vi "Register_ValueCalc.vi"(8 "Index":i32, 9 "ADSxxxx Register Data":T1 {"Base" format="%.0x"; "Item Count" format="%.0x"; "Value" format="%.0x"; "RegMap"."Mask" format="%.0x"; "Default" format="%.0x"; "Register" format="%.0x"}, 11 "Register Controls[]":refnum<vi>[](array[refnum])) -> (2 "Register Value Calculated":u32)   [LabVIEW 2010]
doc: "This VI calculates the register value to write based on the current control values. The VI uses the references to the controls to obtain the current value, and sums the shifted values as appropriate for controls location in the configuration register (provide from register map file).\n\nInputs:\nADSxxxx Register Data - (typdef cluster) contains register information parsed from register map text file\nRegister Controls[] - (control ref array) contains control references to all control with a register cluster control\nIndex - (I32) index to replace # in registers that utilize a common typdef (ie CHxSET)\n\nOutputs:\nRegister Value Calculated - (U32) calculated value of configuration register based on current control settings"
uses:
  Scan RegMap/TYP_ADSxxxx Register.ctl
  Scan RegMap/TYP_RegMap Item.ctl
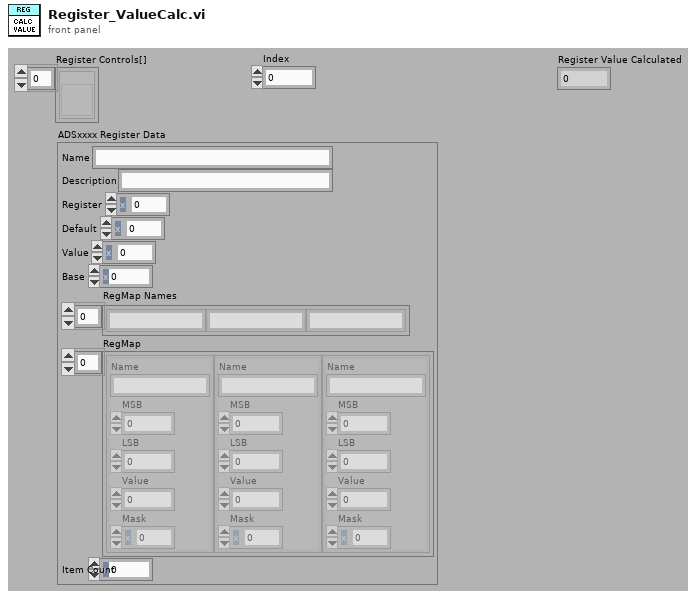
[diagram p1: front panel]
types:
  T1 = typedef "TYP_ADSxxxx Register.ctl" = cluster{"Name":string, "Description":string, "Register":u16, "Default":u16, "Value":u16, "Base":u16, "RegMap Names":string[], "RegMap":T2[], "Item Count":u8}
  T2 = typedef "TYP_RegMap Item.ctl" = cluster{"Name":string, "MSB":u16, "LSB":u16, "Value":u16, "Mask":u16}
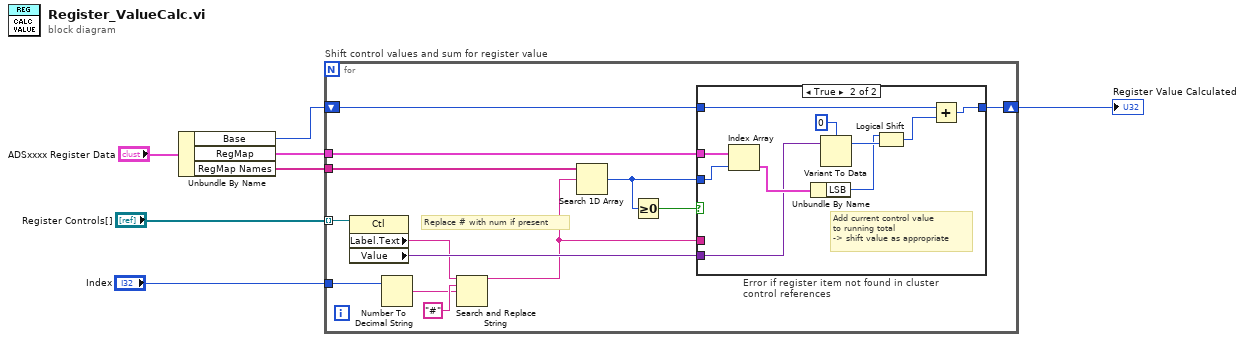
[diagram p0: block diagram]
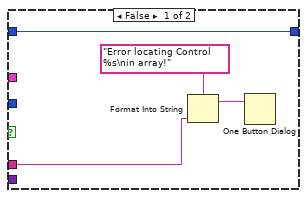
[diagram p2: hidden frame]
diagram:
  n1 = Unbundle By Name("ADSxxxx Register Data") -> ("Base"=w3:u16, "RegMap"=w2:T2[], "RegMap Names"=w5:string[])
  n2 = for "Shift control values and sum for register value" {
    shift-right: [w20] -> w7
    shift-left: w3 -> [w19]
    tunnel: w5 -> [w17]
    tunnel: "Register Controls[]" -> [w16] mode=indexing
    tunnel: w2 -> [w15]
    tunnel: "Index" -> [w9]
    # "Replace # with num if present"
    n3 = property class="Ctl"(reference=w16) -> ("Label.Text"=w12:string, "Value"=w13:variant)  [unwired: 1 in, 2 out]
    n4 = Number To Decimal String(number=w9) -> (decimal integer string=w8:string)  [unwired: 1 in]
    n5 = Search and Replace String(input string=w12, search string="#", replace string=w8) -> (result string=w11:string)  [unwired: 5 in, 3 out]
    n6 = Search 1D Array(1D array=w17, element=w11) -> (index of element=w14:i32)  [unwired: 1 in]
    n7 = Greater Or Equal To 0?(x=w14) -> (x >= 0?=w18:bool)
    n8 = case "Error if register item not found in cluster control references" shown="True" w18 {
      tunnel: [w24 w32] -> w20
      tunnel: w19 -> [w24 w31]
      tunnel: w15 -> [_ w29]
      tunnel: w14 -> [_ w28]
      tunnel: w13 -> [_ w25]
      tunnel: w11 -> [w21 _]
      frame False {
        n9 = Format Into String(format string="Error locating Control %s\nin array!", w21) -> (resulting string=w23:string)  [unwired: 2 in, 1 out]
        n10 = One Button Dialog(message=w23) -> ()  [unwired: 1 in, 1 out]
      }
      frame True {
        # "Add current control value\nto running total\n-> shift value as appropriate"
        n11 = Index Array(array=w29, index=w28) -> (element=w27:T2)
        n12 = Unbundle By Name(w27) -> ("LSB"=w26:u16)
        n13 = Variant To Data(Variant=w25, type=u32 0) -> (data=w33:u32)  [unwired: 1 in, 1 out]
        n14 = Logical Shift(y=w26, x=w33) -> (x << y=w30:u32)
        n15 = Add(x=w31, y=w30) -> (x+y=w32:u32)
      }
    }
  }
  "Register Value Calculated" <- w7
